vi "List Headers.vi"(8 "error in (no error)":errorcluster, 11 "HTTP Client Advanced in":refnum<class "HTTP Client Advanced.lvclass">) -> (0 "error out":errorcluster, 2 "headers":string, 3 "HTTP Client Advanced out":refnum<class "HTTP Client Advanced.lvclass">)   [LabVIEW 2021, in "HTTP Client Advanced.lvclass"]
uses:
  HTTP Client Advanced.lvclass
  HTTP Client Advanced.lvclass/HTTP Client Advanced.ctl
  <vilib>/NI/Advanced HTTP Client/Session.lvclass
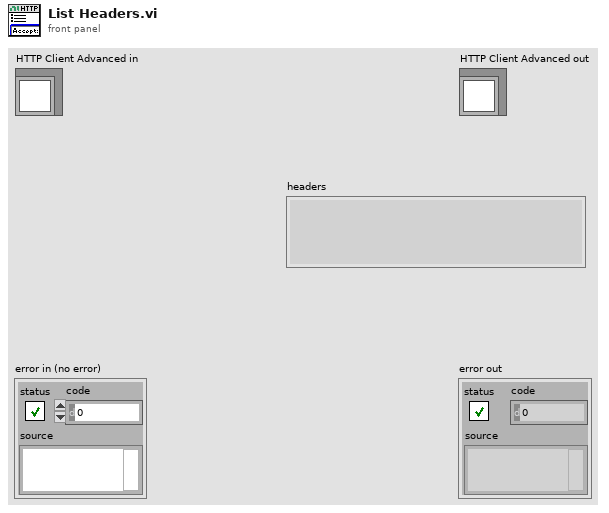
[diagram p1: front panel]
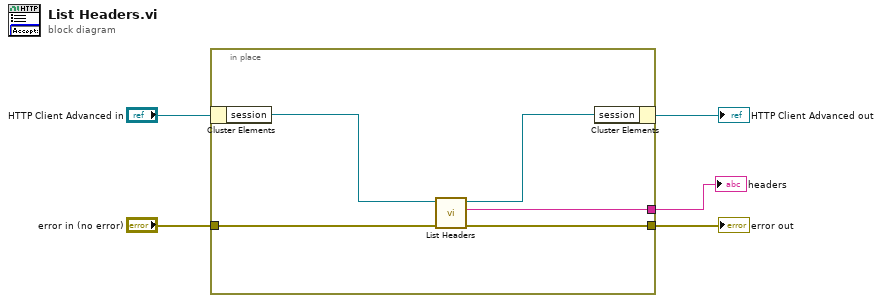
[diagram p0: block diagram]
diagram:
  n1 = in-place {
    in-place-border: "error in (no error)" -> [w10]
    in-place-border: [w9] -> w4
    in-place-border: [w6] -> w1
    n2 = in-place-cluster #1("HTTP Client Advanced in") -> ("session"=w7:refnum<class "Session.lvclass">)
    n3 = call <vilib>:"List Headers.vi"("error in"=w10, "session in"=w7) -> ("error out"=w9:errorcluster, "headers"=w6:string, "session out"=w8:refnum<class "Session.lvclass">)  [unwired: 7 in]
    n4 = in-place-cluster #1("session"=w8) -> (→"HTTP Client Advanced out":refnum<class "HTTP Client Advanced.lvclass">)
  }
  "error out" <- w4
  "headers" <- w1
